vi "Resideo Error Mapping.vi"(11 "Error Code Number":string) -> (3 "Error Status":string)   [LabVIEW 2020]
uses:
  <vilib>/Utility/error.llb/whitespace.ctl
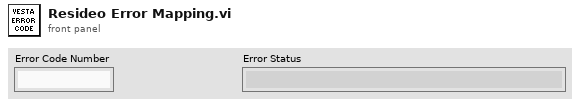
[diagram p1: front panel]
types:
  T1 = typedef "whitespace.ctl" = u16
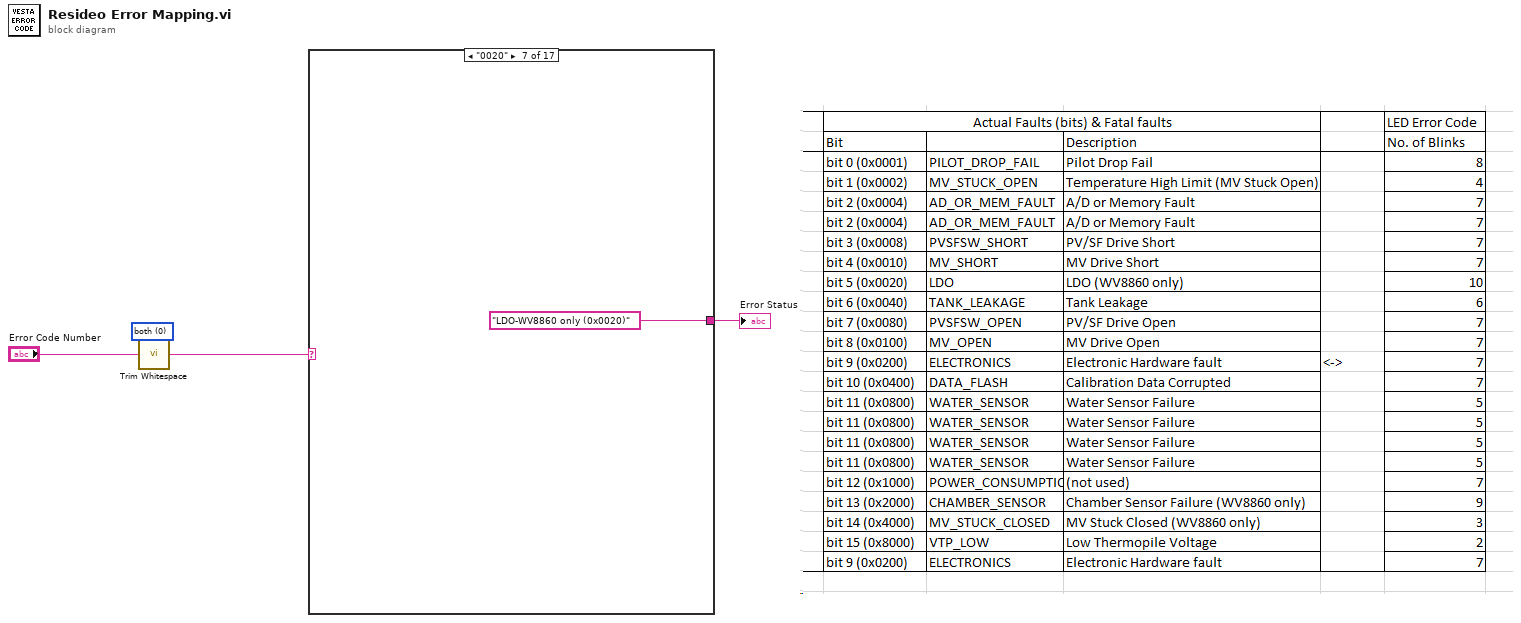
[diagram p0: block diagram]
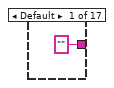
[diagram p2: hidden frame]
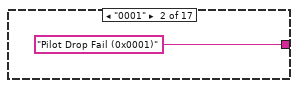
[diagram p3: hidden frame]
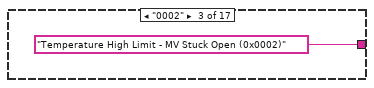
[diagram p4: hidden frame]
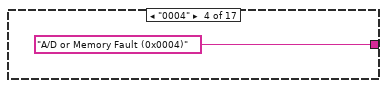
[diagram p5: hidden frame]
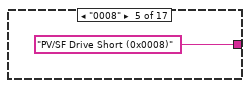
[diagram p6: hidden frame]
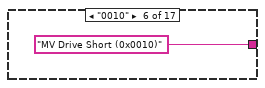
[diagram p7: hidden frame]
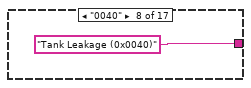
[diagram p8: hidden frame]
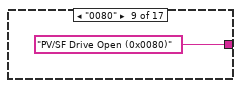
[diagram p9: hidden frame]
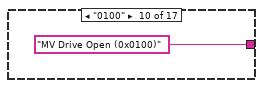
[diagram p10: hidden frame]
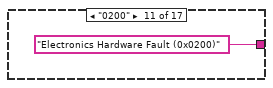
[diagram p11: hidden frame]
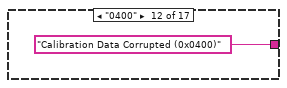
[diagram p12: hidden frame]
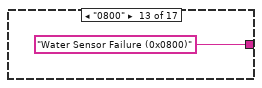
[diagram p13: hidden frame]
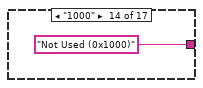
[diagram p14: hidden frame]
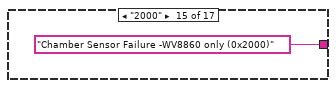
[diagram p15: hidden frame]
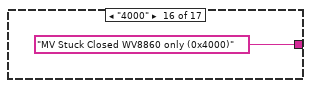
[diagram p16: hidden frame]
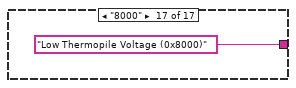
[diagram p17: hidden frame]
diagram:
  w3 = T1 0 items=["both", "start of string", "end of string"] ("location (both)")
  n1 = call <vilib>:"Trim Whitespace.vi"("string"="Error Code Number", "location (both)"=w3) -> ("trimmed string"=w2:string)
  n2 = case shown="\"0020\"" w2 {
    tunnel: ["" "Pilot Drop Fail (0x0001)" "Temperature High Limit - MV Stuck Open (0x0002)" "A/D or Memory Fault (0x0004)" "PV/SF Drive Short (0x0008)" "MV Drive Short (0x0010)" "LDO-WV8860 only (0x0020)" "Tank Leakage (0x0040)" "PV/SF Drive Open (0x0080)" "MV Drive Open (0x0100)" "Electronics Hardware Fault (0x0200)" "Calibration Data Corrupted (0x0400)" "Water Sensor Failure (0x0800)" "Not Used (0x1000)" "Chamber Sensor Failure -WV8860 only (0x2000)" "MV Stuck Closed WV8860 only (0x4000)" "Low Thermopile Voltage (0x8000)"] -> w1
    frame Default {
    }
    frame "0001" {
    }
    frame "0002" {
    }
    frame "0004" {
    }
    frame "0008" {
    }
    frame "0010" {
    }
    frame "0020" {
    }
    frame "0040" {
    }
    frame "0080" {
    }
    frame "0100" {
    }
    frame "0200" {
    }
    frame "0400" {
    }
    frame "0800" {
    }
    frame "1000" {
    }
    frame "2000" {
    }
    frame "4000" {
    }
    frame "8000" {
    }
  }
  "Error Status" <- w1
